vi "GenerateAttackablePosition_Pawn.vi"(1 "Black/White (T/F)":bool, 2 "Board":i32[][](array[numeric])=[[-3, -5, -4, -1, -2, -4, -5, -3], [-6, -6, -6, -6, -6, -6, -6, -6], [0, 0, 0, 0, 0, 0, 0, 0], [0, 0, 0, 0, 0, 0, 0, 0], [0, 0, 0, 0, 0, 0, 0, 0], [0, 0, 0, 0, 0, 0, 0, 0], [6, 6, 6, 6, 6, 6, 6, 6], [3, 5, 4, 1, 2, 4, 5, 3]], 3 "pieceIndex":i32) -> (0 "AttackablePosition":bool[][](array[boolean]))   [LabVIEW 2014]
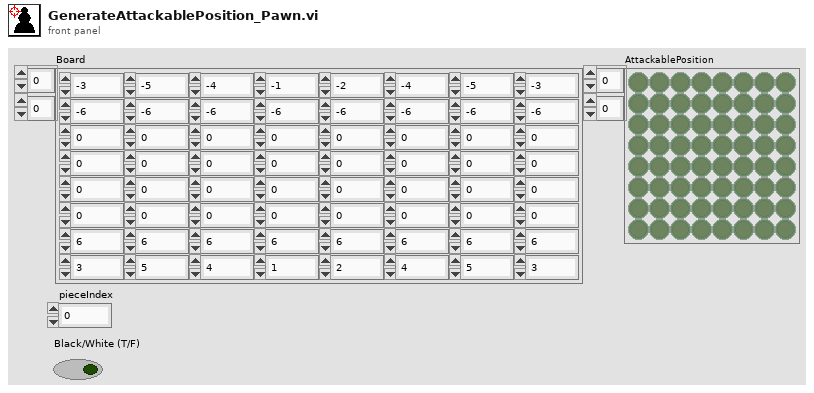
[diagram p1: front panel]
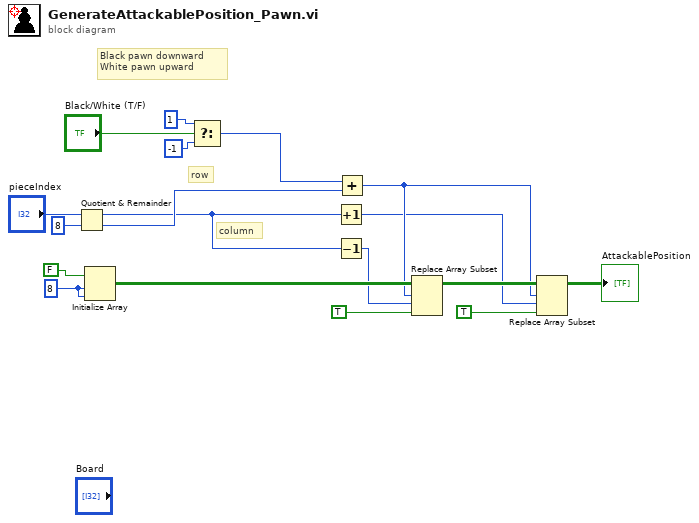
[diagram p0: block diagram]
diagram:
  w16 = 8 ("dimension size")
  # "Black pawn downward\nWhite pawn upward"
  # "column"
  # "row"
  n1 = Quotient & Remainder(x="pieceIndex", y=8) -> (x-y*floor(x/y)=w9:i32, floor(x/y)=w11:i32)
  n2 = Initialize Array(FALSE, w16, w16) -> (w8:bool[][])
  n3 = Select(t=1, s="Black/White (T/F)", f=-1) -> (s? t:f=w10:i32)
  n4 = Increment(x=w9) -> (x+1=w2:i32)
  n5 = Decrement(x=w9) -> (x-1=w7:i32)
  n6 = Add(x=w10, y=w11) -> (x+y=w3:i32)
  n7 = Replace Array Subset(array=w8, new element=TRUE, index (row)=w3, index (col)=w7) -> (w4:bool[][])
  n8 = Replace Array Subset(array=w4, new element=TRUE, index (row)=w3, index (col)=w2) -> (→"AttackablePosition":bool[][])
